vi "AVS_Main.vi"() -> ()   [LabVIEW 2016]
uses:
  Instance           5 16Saved   AVS_Main .vi
  Instance           6 16Saved   AVS_Main .vi
  Instance           4 16Saved   AVS_Main .vi
  <vilib>/express/express arith-compare/Formula/XNode/ExpressFormulaBlockNode.xnode
panel:
  out "a_hDevice":i32
  out "StartTime":u32
  out "XY Graph":cluster{"Y":dbl[], "Y":dbl[]}[](graph)
  out "LastScanTime":dbl caption="Last scan in [ms]" format="%#4.2f"
  out "AvgTimePerScan":dbl caption="Avg Time /Scan [ms]" format="%#4.2f"
  out "Failures":dbl caption="Nr Of Failures" format="%#.0f"
  out "PerformedScans":dbl caption="Nr Of Scans" format="%#.0f"
  out "TotalTime":dbl caption="Time Since Start [s]" format="%#.1f"
  in  "StopMeasurement":bool
  out "Status":string
  in  "StartMeasurement":bool caption="Start Measurement"
  in  "NrOfScans":i16 caption="Nr Of Scans"
  in  "RamSpectra":u16 caption="Spectra stored to RAM"
  in  "LaserWavelenght":sgl caption="Laser Wavelenght [nm]" format="%.2f"
  in  "LaserWidth":u32 caption="Laser Width [ns]"
  in  "LaserDelay":u32 caption="Laser Delay [ns]"
  in  "FlashesPerScan":u16 caption="Flashes per Scan"
  in  "SmoothModel":u8 caption="Model"
  in  "SmoothPix":u16 caption="Nr Of Pixels"
  in  "EnableDarkCorrection":bool caption="Enable"
  in  "DarkHist":u8 caption="%"
  in  "SatDetection":u8 caption="Saturation detection"
  in  "NrOfAVG":u32 caption="Number of averages"
  in  "IntDelay":dbl caption="Integration delay [ns]" min=-20.0 format="%#.0f"
  in  "IntTime":sgl caption="Integration time [ms]" format="%.2f"
  in  "StartPixel":u16 caption="Start pixel"
  in  "StopPixel":u16 caption="Stop pixel"
  in  "Trigger type":enum32{"Radio Selection 1", "Radio Selection 2"}(radio)
  in  "Trigger source":enum32{"Radio Selection 1", "Radio Selection 2"}(radio)
  in  "Trigger mode":T1(radio)
  out "DllVersion":string caption="AS5216 Dll Version"
  out "FWVersion":string caption="AS5216 FW Version"
  out "FPGAVersion":string caption="FPGA Version"
  out "NrOfPixel":u16 caption="Nr Of Pixels"
  out "Detector":string
  in  "Exit":bool
  in  "WriteMeasToEEProm":bool
  in  "ReadMeasFromEEProm":bool
  in  "AnalogIO":bool
  in  "DigitalIO":bool
  # "Dark Correction Settings"
  # "Measure"
  # "(-1 = infinite)"
  # "Smoothing Settings"
  # "Control Settings"
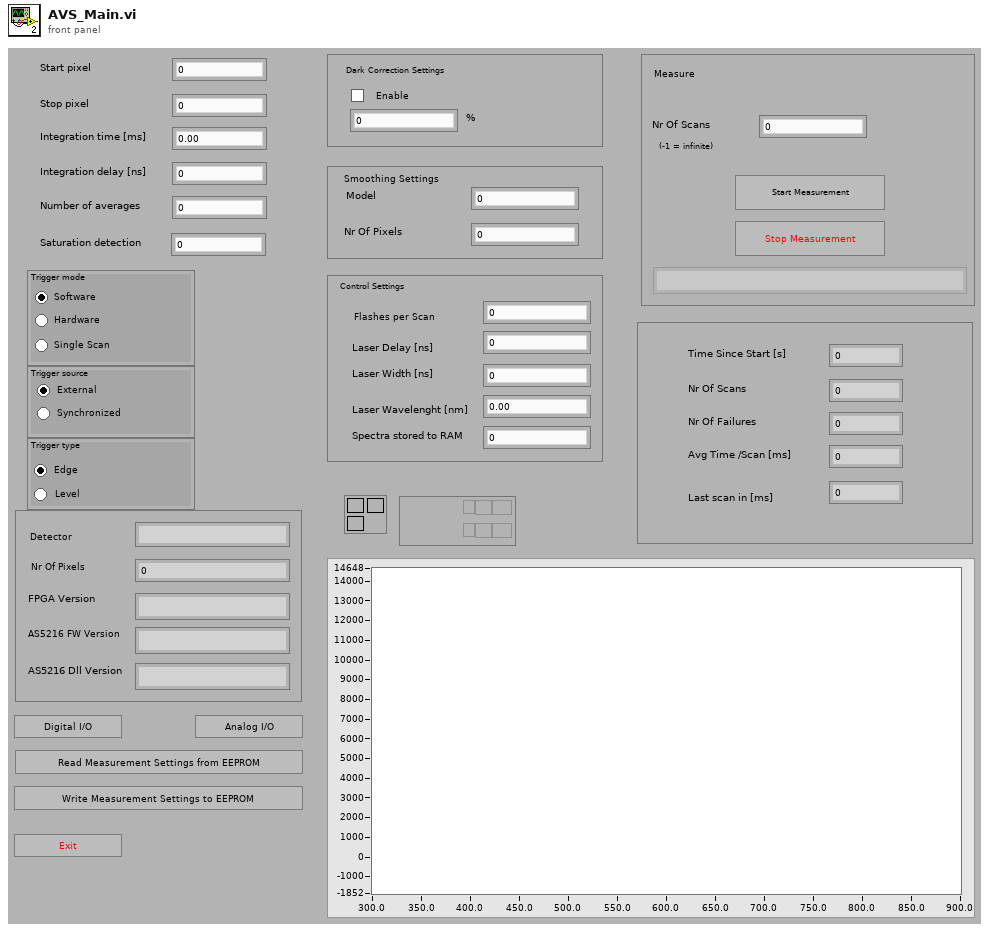
[diagram p1: front panel]
types:
  T1 = enum32{"Radio Selection 1", "Radio Selection 2", "Radio Selection 3"}
  T2 = cluster{"Len":u16, "ConfigVersion":u16, "UserFriendlyId":u8[], "DetectorType":cluster{"SensorType":u8, "NrPixels":u16, "Fit":sgl[], "NLEnable":u8, "NLCorrect":dbl[], "LowNLCounts":dbl, "HighNLCounts":dbl, "Gain":sgl[], "Reserved":sgl, "Offset":sgl[], "Extern Offset":sgl, "DefectivePixels":u16[]}, "IrradianceType":cluster{"SpectrumCalibrationType":cluster{"SmoothingType":cluster{"m_SmoothPix":u16, "SmoothModel":u8}, "CalInttime":sgl, "CalibConvers":sgl[]}, "CalibrationType":u8, "FiberDiameter":i32}, "SpectrumCalibrationType":cluster{"SmoothingType":cluster{"m_SmoothPix":u16, "SmoothModel":u8}, "CalInttime":sgl, "CalibConvers":sgl[]}, "SpectrumCorrectionType":sgl[], "StandAloneType":cluster{"StandAloneType":u8, "MeasConfigType":cluster{"StartPixel":u16, "StopPixel":u16, "IntegrationTime":sgl, "IntegrationDelay":u32, "NrAverages":u32, "DarkCorrectionType":cluster{"Enable CorDynDark":u8, "ForgetPercentage":u8}, "SmoothingType":cluster{"SmoothPix":u16, "SmoothModel":u8}, "SatDetection":u8, "TriggerType":cluster{"Trigger Mode":u8, "Trigger Source":u8, "Trigger SourceType":u8}, "ControlSettingsType":cluster{"StrobeControl":u16, "LaserDelay":u32, "LaserWidth":u32, "LaserWaveLength":sgl, "StoreToRam":u16}}, "Nmsr":i16}, "DynamicStorageType":cluster{"Nmsr":i32, "Reserved":u8[]}, "TempSensorType":sgl[], "TecControlType":cluster{"Enable":u8, "Setpoint":sgl, "Fit[NR_DAC_POL_COEF]":sgl[]}, "ProcessControlType":cluster{"AnalogLow":sgl[], "AnalogHigh":sgl[], "DigitalLow":sgl[], "DigitalHigh":sgl[]}, "EthernetSettingsType":cluster{"IpAddr":u32, "NetMask":u32, "Gateway":u32, "DhcpEnabled":u8, "TcpPort":u16, "LinkStatus":u8}, "Reserved":u8[]}
  T3 = cluster{"StartPixel":u16, "StopPixel":u16, "IntegrationTime":sgl, "IntegrationDelay":u32, "NrAverages":u32, "DarkCorrectionType":cluster{"Enable CorDynDark":u8, "ForgetPercentage":u8}, "SmoothingType":cluster{"SmoothPix":u16, "SmoothModel":u8}, "SatDetection":u8, "TriggerType":cluster{"Trigger Mode":u8, "Trigger Source":u8, "Trigger SourceType":u8}, "ControlSettingsType":cluster{"StrobeControl":u16, "LaserDelay":u32, "LaserWidth":u32, "LaserWaveLength":sgl, "StoreToRam":u16}}
  T4 = cluster{"FlashesPerScan":u16, "Result":u32, "Result":u32, "LaserWavelenght":sgl, "RamSpectra":u16}
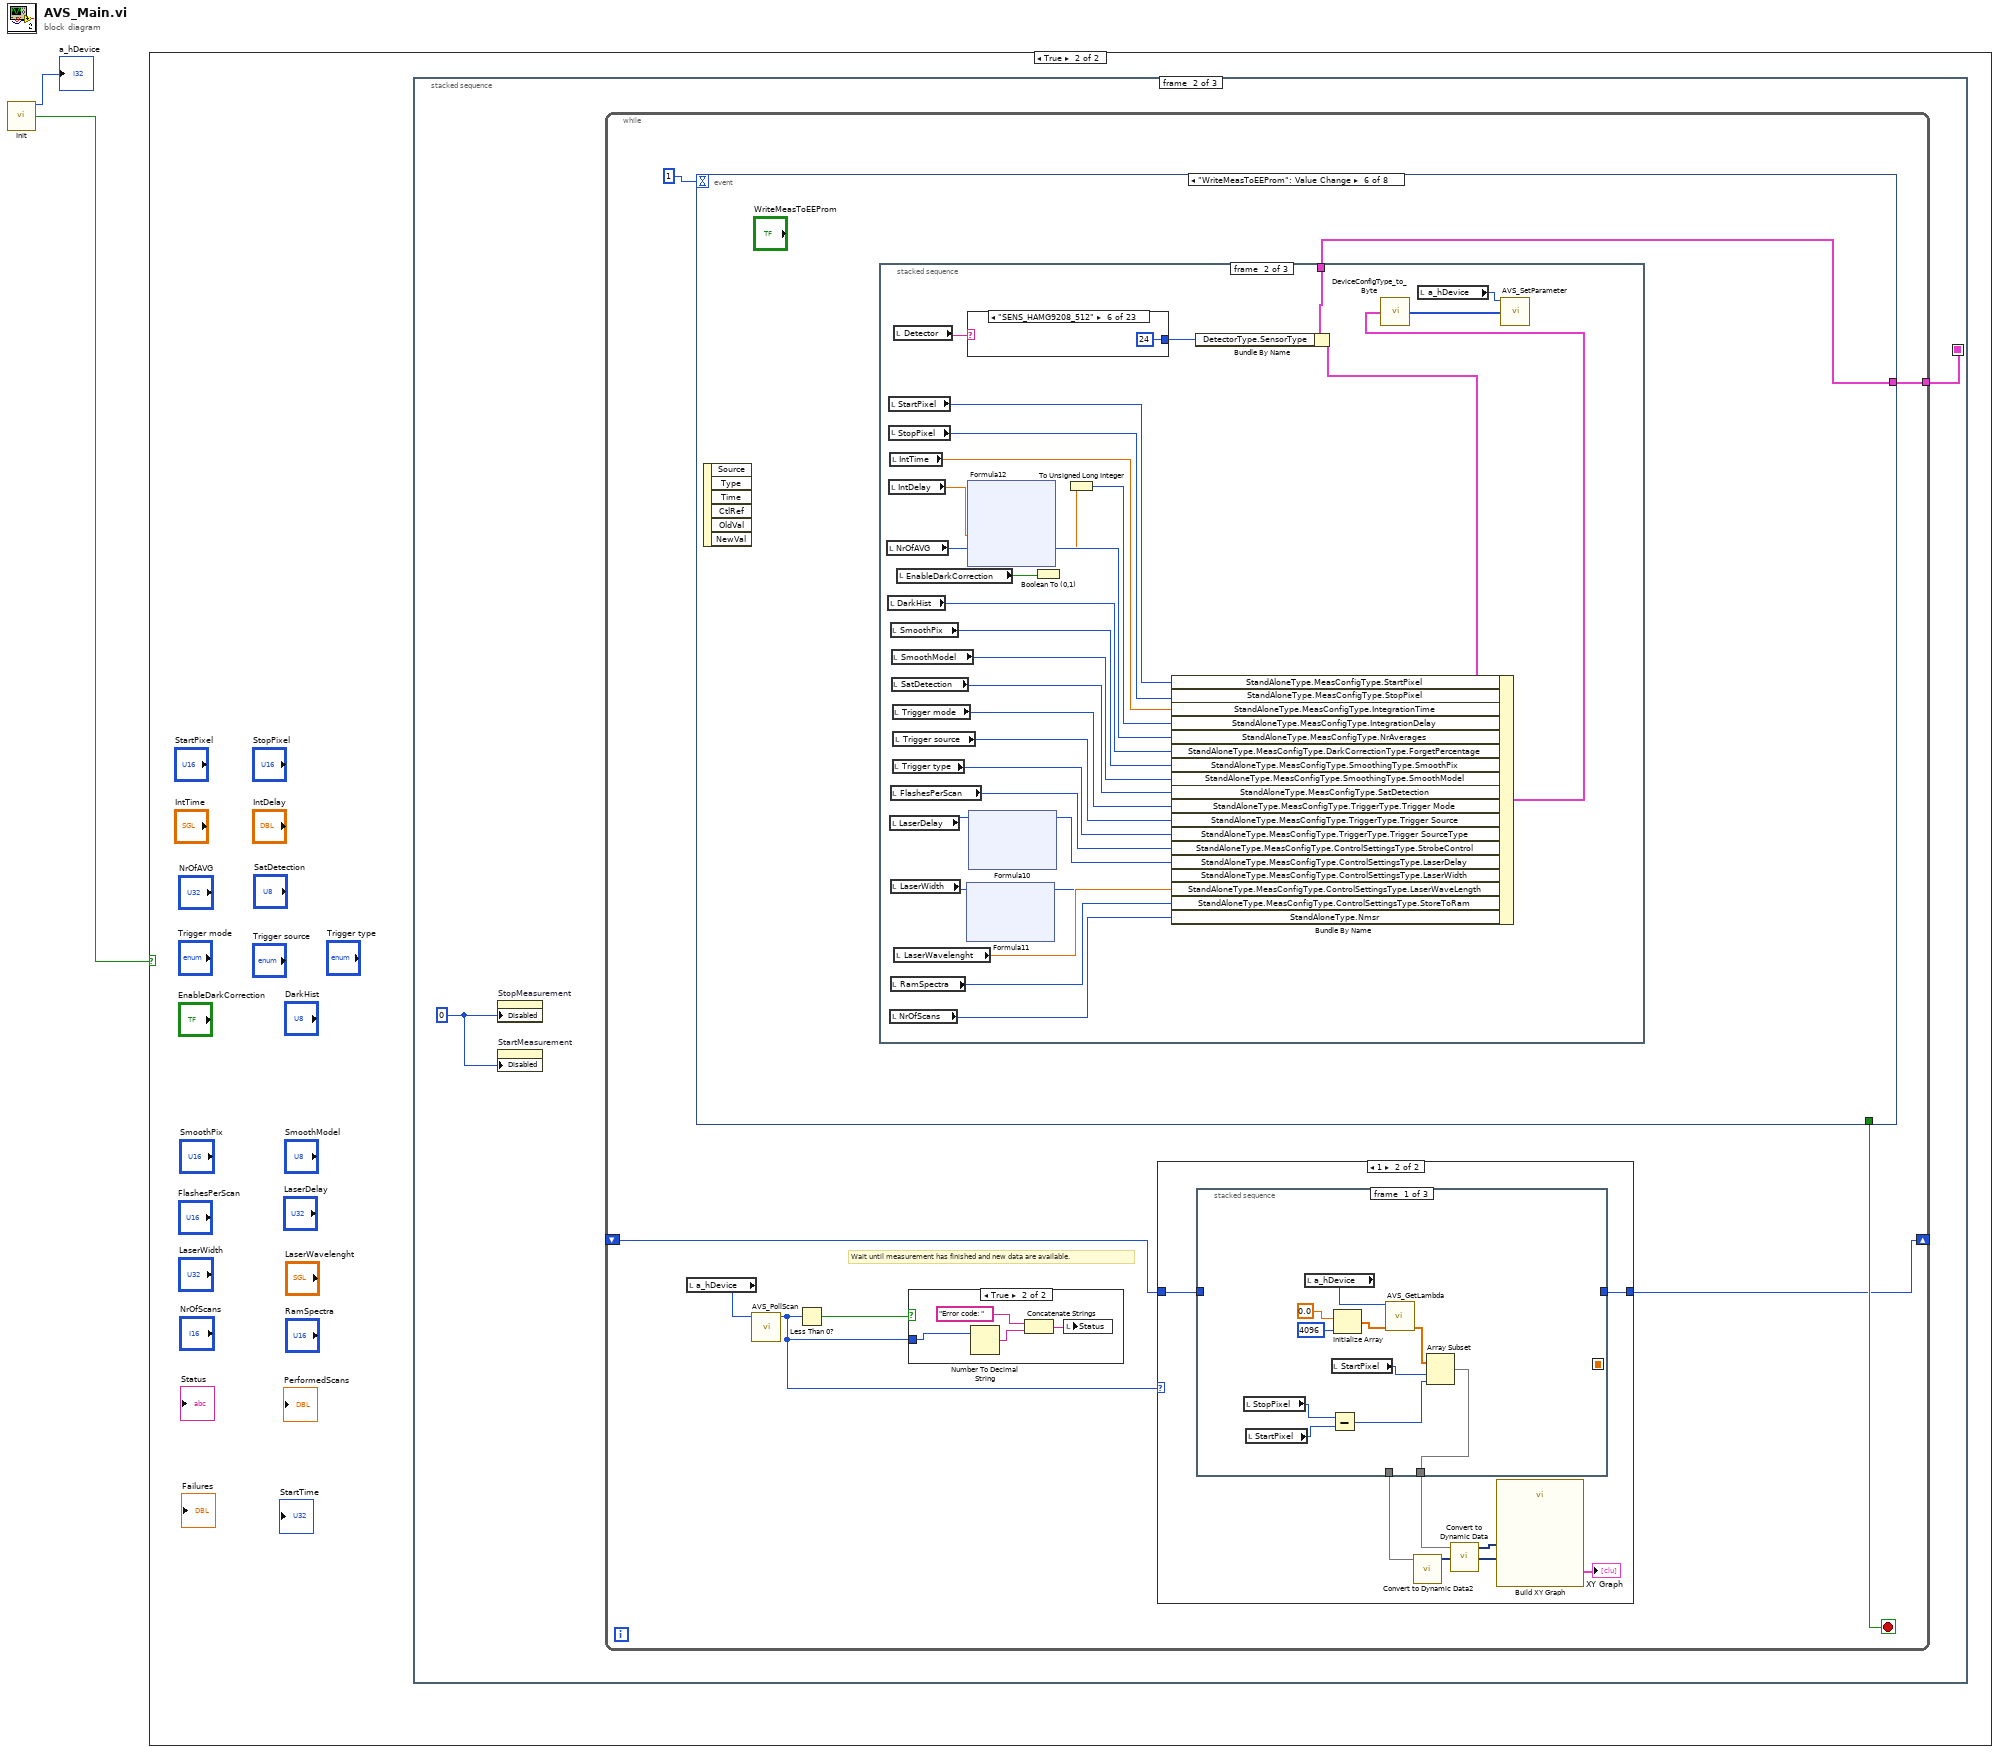
[diagram p0: block diagram]
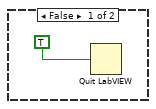
[diagram p2: hidden frame]
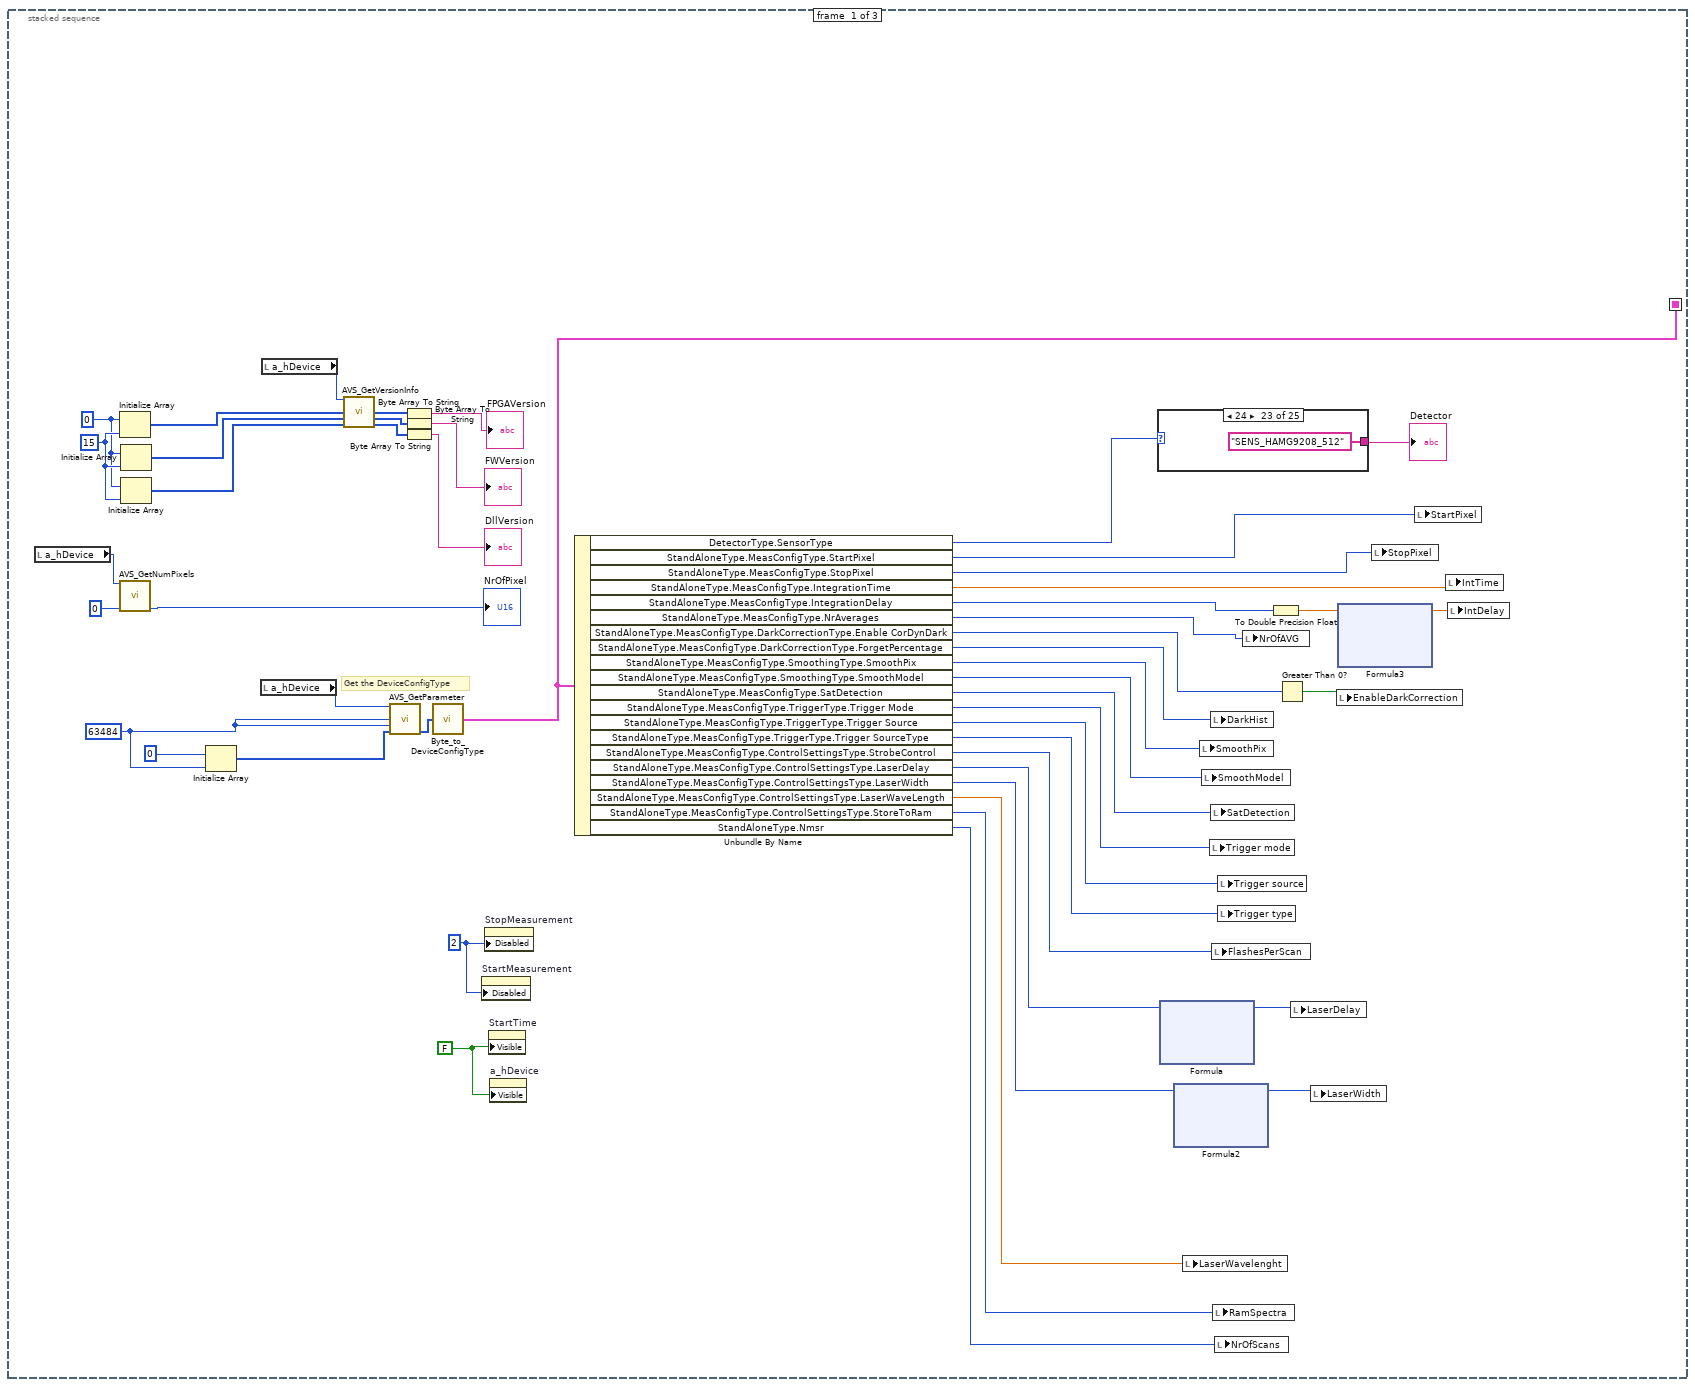
[diagram p3: hidden frame]
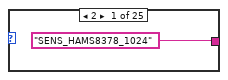
[diagram p4: hidden frame]
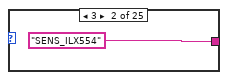
[diagram p5: hidden frame]
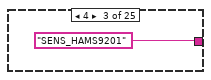
[diagram p6: hidden frame]
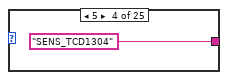
[diagram p7: hidden frame]
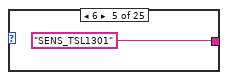
[diagram p8: hidden frame]
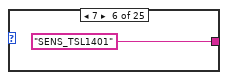
[diagram p9: hidden frame]
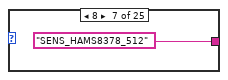
[diagram p10: hidden frame]
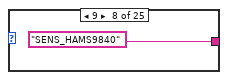
[diagram p11: hidden frame]
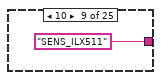
[diagram p12: hidden frame]
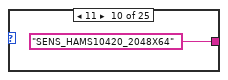
[diagram p13: hidden frame]
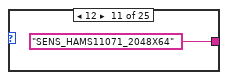
[diagram p14: hidden frame]
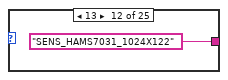
[diagram p15: hidden frame]
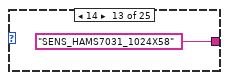
[diagram p16: hidden frame]
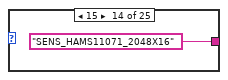
[diagram p17: hidden frame]
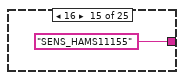
[diagram p18: hidden frame]
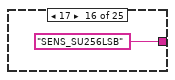
[diagram p19: hidden frame]
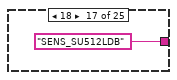
[diagram p20: hidden frame]
diagram:
  n1 = call "Init.vi"() -> ("a_hDevice"=→"a_hDevice":i32, "Available"=w2:bool)  [unwired: 14 in]
  n2 = case shown="True" w2 {
    frame False {
      n3 = Quit LabVIEW(quit? (T)=TRUE) -> ()
    }
    frame True {
      n4 = stacked-sequence {
        seq-local: [w9 _ _] -> [_ w102 _]
        frame #0 {
          w4 = FALSE
          w40 = u8 2 ("Disabled")
          w39 = u16 63484 ("a_pNumPixelsInput")
          w44 = u8 0
          w45 = u16 15 ("a_pNumPixelsInput")
          # "Get the DeviceConfigType"
          n5 = local read "a_hDevice"() -> (w8:i32)
          n6 = Initialize Array(w44, w45) -> (w48:u8[])
          n7 = call "AVS_GetNumPixels.vi"("a_hDevice"=w8, "a_pNumPixels"=u16 0 ("a_pNumPixelsInput")) -> ("a_pNumPixels"=→"NrOfPixel":u16)  [unwired: 12 in, 1 out]
          n8 = Initialize Array(w44, w45) -> (w47:u8[])
          n9 = Initialize Array(w44, w45) -> (w46:u8[])
          n10 = Initialize Array(u8 0, w39) -> (w38:u8[])
          n11 = local read "a_hDevice"() -> (w6:i32)
          n12 = local read "a_hDevice"() -> (w7:i32)
          n13 = call "AVS_GetVersionInfo.vi"("a_hDevice"=w7, "a_pFPGAVersion"=w48, "a_pFirmwareVersion"=w47, "a_pDLLVersion"=w46) -> ("a_pFPGAVersion"=w52:i8[], "a_pFirmwareVersion"=w51:i8[], "a_pDLLVersion"=w50:i8[])  [unwired: 8 in, 1 out]
          n14 = call "AVS_GetParameter.vi"("a_hDevice"=w6, "a_Size"=w39, "RequiredSizeInput"=w39, "DeviceParm"=w38) -> ("DeviceParam"=w37:u8[])  [unwired: 9 in, 2 out]
          n15 = Byte Array To String(unsigned byte array=w52) -> (string=→"FPGAVersion":string)
          n16 = Byte Array To String(unsigned byte array=w51) -> (string=→"FWVersion":string)
          n17 = Byte Array To String(unsigned byte array=w50) -> (string=→"DllVersion":string)
          n18 = call "Byte_to_DeviceConfigType.vi"("Byte Array"=w37) -> ("output cluster"=w9:T2)  [unwired: 4 in]
          n19 = property on="StartMeasurement" class="Bool"("Disabled"=w40) -> ()  [unwired: 2 in, 2 out]
          n20 = property on="StopMeasurement" class="Bool"("Disabled"=w40) -> ()  [unwired: 2 in, 2 out]
          n21 = property on="StartTime" class="DigNum (strict)"("Visible"=w4) -> ()  [unwired: 2 in, 2 out]
          n22 = property on="a_hDevice" class="DigNum (strict)"("Visible"=w4) -> ()  [unwired: 2 in, 2 out]
          n23 = Unbundle By Name(w9) -> ("DetectorType.SensorType"=w34:u8, "StandAloneType.MeasConfigType.StartPixel"=w33:u16, "StandAloneType.MeasConfigType.StopPixel"=w32:u16, "StandAloneType.MeasConfigType.IntegrationTime"=w31:sgl, "StandAloneType.MeasConfigType.IntegrationDelay"=w30:u32, "StandAloneType.MeasConfigType.NrAverages"=w29:u32, "StandAloneType.MeasConfigType.DarkCorrectionType.Enable CorDynDark"=w27:u8, "StandAloneType.MeasConfigType.DarkCorrectionType.ForgetPercentage"=w26:u8, "StandAloneType.MeasConfigType.SmoothingType.SmoothPix"=w25:u16, "StandAloneType.MeasConfigType.SmoothingType.SmoothModel"=w24:u8, "StandAloneType.MeasConfigType.SatDetection"=w23:u8, "StandAloneType.MeasConfigType.TriggerType.Trigger Mode"=w22:u8, "StandAloneType.MeasConfigType.TriggerType.Trigger Source"=w21:u8, "StandAloneType.MeasConfigType.TriggerType.Trigger SourceType"=w20:u8, "StandAloneType.MeasConfigType.ControlSettingsType.StrobeControl"=w19:u16, "StandAloneType.MeasConfigType.ControlSettingsType.LaserDelay"=w18:u32, "StandAloneType.MeasConfigType.ControlSettingsType.LaserWidth"=w17:u32, "StandAloneType.MeasConfigType.ControlSettingsType.LaserWaveLength"=w16:sgl, "StandAloneType.MeasConfigType.ControlSettingsType.StoreToRam"=w15:u16, "StandAloneType.Nmsr"=w14:i16)
          n24 = case shown="24" w34 {
            tunnel: ["SENS_HAMS8378_1024" ("String") "SENS_ILX554" ("String") "SENS_HAMS9201" ("String") "SENS_TCD1304" ("String") "SENS_TSL1301" ("String") "SENS_TSL1401" ("String") "SENS_HAMS8378_512" ("String") "SENS_HAMS9840" ("String") "SENS_ILX511" ("String") "SENS_HAMS10420_2048X64" ("String") "SENS_HAMS11071_2048X64" ("String") "SENS_HAMS7031_1024X122" ("String") "SENS_HAMS7031_1024X58" ("String") "SENS_HAMS11071_2048X16" ("String") "SENS_HAMS11155" ("String") "SENS_SU256LSB" ("String") "SENS_SU512LDB" ("String") "unknown" ("String") "unknown" ("String") "SENS_HAMS11638" ("String") "SENS_HAMS11639" ("String") "SENS_HAMS12443" ("String") "SENS_HAMG9208_512" ("String") "unknown" ("String") "SENS_HAMS8378_256" ("String")] -> w5
            frame 2 {
            }
            frame 3 {
            }
            frame 4 {
            }
            frame 5 {
            }
            frame 6 {
            }
            frame 7 {
            }
            frame 8 {
            }
            frame 9 {
            }
            frame 10 {
            }
            frame 11 {
            }
            frame 12 {
            }
            frame 13 {
            }
            frame 14 {
            }
            frame 15 {
            }
            frame 16 {
            }
            frame 17 {
            }
            frame 18 {
            }
            frame 19 {
            }
            frame 20 {
            }
            frame 21 {
            }
            frame 22 {
            }
            frame 23 {
            }
            frame 24 {
            }
            frame Default {
            }
            frame 1 {
            }
          }
          "Detector" <- w5
          n25 = xnode "Formula"("X1"=w18) -> ("Result"=w42:u32)  [unwired: 1 in, 1 out]
          n26 = xnode "Formula2"("X1"=w17) -> ("Result"=w41:u32)  [unwired: 1 in, 1 out]
          n27 = local write "LaserWavelenght"(w16) -> ()
          n28 = local write "SmoothPix"(w25) -> ()
          n29 = local write "SmoothModel"(w24) -> ()
          n30 = local write "Trigger mode"(w22) -> ()
          n31 = local write "DarkHist"(w26) -> ()
          n32 = local write "SatDetection"(w23) -> ()
          n33 = local write "FlashesPerScan"(w19) -> ()
          n34 = local write "RamSpectra"(w15) -> ()
          n35 = local write "NrOfScans"(w14) -> ()
          n36 = local write "Trigger source"(w21) -> ()
          n37 = local write "Trigger type"(w20) -> ()
          n38 = local write "NrOfAVG"(w29) -> ()
          n39 = To Double Precision Float(number=w30) -> (double precision float=w36:dbl)
          n40 = Greater Than 0?(x=w27) -> (x > 0?=w28:bool)
          n41 = local write "LaserDelay"(w42) -> ()
          n42 = local write "LaserWidth"(w41) -> ()
          n43 = local write "EnableDarkCorrection"(w28) -> ()
          n44 = xnode "Formula3"("X1"=w36) -> ("Result"=w35:dbl)  [unwired: 1 in, 1 out]
          n45 = local write "StopPixel"(w32) -> ()
          n46 = local write "StartPixel"(w33) -> ()
          n47 = local write "IntTime"(w31) -> ()
          n48 = local write "IntDelay"(w35) -> ()
        }
        frame #1 {
          w103 = u8 0 ("Disabled")
          n49 = property on="StopMeasurement" class="Bool"("Disabled"=w103) -> ()  [unwired: 2 in, 2 out]
          n50 = property on="StartMeasurement" class="Bool"("Disabled"=w103) -> ()  [unwired: 2 in, 2 out]
          n51 = while {
            tunnel: w102 -> [w107]
            shift-right: [w106] -> _
            shift-left: _ -> [w105]
            stop <- w111 stop-if-true
            # "Wait until measurement has finished and new data are available."
            n52 = local read "a_hDevice"() -> (w109:i32)
            n53 = event shown="[5] \"WriteMeasToEEProm\": Value Change" {
              selector: _ -> [_ _ _ _ _ _ _ _]
              dyn-events: _ -> [_ _ _ _ _ _ _ _]
              timeout: 1 -> [_ _ _ _ _ _ _ _]
              tunnel: [_ _ _ _ _ _ _ "Exit"] -> w111
              tunnel: w107 -> [_ _ _ _ _ w320 _ _]
              event Timeout {
                n54 = event-data() -> ()  [unwired: 1 in, 2 out]
              }
              event "StartMeasurement": Value Change {
                w190 = T3 {"StartPixel"=0, "StopPixel"=0, "IntegrationTime"=0.0, "IntegrationDelay"=0, "NrAverages"=0, "DarkCorrectionType"={"Enable CorDynDark"=0, "ForgetPercentage"=0}, "SmoothingType"={"SmoothPix"=0, "SmoothModel"=0}, "SatDetection"=0, "TriggerType"={"Trigger Mode"=0, "Trigger Source"=0, "Trigger SourceType"=0}, "ControlSettingsType"={"StrobeControl"=0, "LaserDelay"=0, "LaserWidth"=0, "LaserWaveLength"=0.0, "StoreToRam"=0}}  # MeasConfigType
                w172 = u8 2 ("Disabled")
                w196 = 0.0 ("Failures")
                # "StartMeas:\n1: Prepares measurement on the spectrometer \nusing the specified measurement configuration. \n2: Start measurement"
                n55 = event-data() -> ()  [unwired: 1 in, 6 out]
                n56 = local read "EnableDarkCorrection"() -> (w197:bool)
                n57 = local read "SmoothModel"() -> (w185:u8)
                n58 = local read "Trigger mode"() -> (w199:T1)
                n59 = local read "FlashesPerScan"() -> (w173:u16)
                n60 = local read "SmoothPix"() -> (w186:u16)
                n61 = local read "SatDetection"() -> (w182:u8)
                n62 = local read "RamSpectra"() -> (w177:u16)
                n63 = local read "Trigger source"() -> (w200:enum32{"Radio Selection 1", "Radio Selection 2"})
                n64 = local read "LaserWavelenght"() -> (w176:sgl)
                n65 = local read "DarkHist"() -> (w188:u8)
                n66 = local read "Trigger type"() -> (w198:enum32{"Radio Selection 1", "Radio Selection 2"})
                n67 = local read "LaserDelay"() -> (w192:u32)
                n68 = local read "LaserWidth"() -> (w191:u32)
                n69 = local read "StartPixel"() -> (w204:u16)
                n70 = local read "StopPixel"() -> (w203:u16)
                n71 = local read "IntTime"() -> (w202:sgl)
                n72 = local read "NrOfAVG"() -> (w205:u32)
                n73 = local read "IntDelay"() -> (w193:dbl)
                n74 = xnode "Formula6"("X1"=w191) -> ("Result"=w175:u32)  [unwired: 1 in, 1 out]
                n75 = xnode "Formula5"("X1"=w192) -> ("Result"=w174:u32)  [unwired: 1 in, 1 out]
                n76 = Boolean To (0,1)(Boolean=w197) -> (0, 1=w201:i16)
                n77 = Bundle("SmoothPix"=w186, "SmoothModel"=w185) -> (w184:cluster{"SmoothPix":u16, "SmoothModel":u8})  [unwired: 1 in]
                n78 = xnode "Formula4"("X1"=w193) -> ("Result"=w194:dbl)  [unwired: 1 in, 1 out]
                n79 = To Unsigned Byte Integer(number=w201) -> (unsigned 8bit integer=w189:u8)
                n80 = To Unsigned Byte Integer(number=w200) -> (unsigned 8bit integer=w180:u8)
                n81 = Bundle(w189, "DarkHist"=w188) -> (w187:cluster{u8, "DarkHist":u8})  [unwired: 1 in]
                n82 = To Unsigned Byte Integer(number=w199) -> (unsigned 8bit integer=w183:u8)
                n83 = To Unsigned Byte Integer(number=w198) -> (unsigned 8bit integer=w181:u8)
                n84 = To Unsigned Long Integer(number=w194) -> (unsigned 32bit integer=w195:u32)
                n85 = Bundle("FlashesPerScan"=w173, "Result"=w174, "Result"=w175, "LaserWavelenght"=w176, "RamSpectra"=w177) -> (w178:T4)  [unwired: 1 in]
                n86 = Bundle(w183, w180, w181) -> (w179:cluster{u8, u8, u8})  [unwired: 1 in]
                n87 = Bundle(cluster=w190, "StartPixel"=w204, "StopPixel"=w203, "IntegrationTime"=w202, "IntegrationDelay"=w195, "NrAverages"=w205, "DarkCorrectionType"=w187, "SmoothingType"=w184, "SatDetection"=w182, "TriggerType"=w179, "ControlSettingsType"=w178) -> (w206:T3)
                n88 = local write "Failures"(w196) -> ()
                n89 = local write "TotalTime"(w196) -> ()
                n90 = local write "PerformedScans"(w196) -> ()
                n91 = local write "AvgTimePerScan"(w196) -> ()
                n92 = local write "LastScanTime"(w196) -> ()
                n93 = local read "NrOfScans"() -> (w168:i16)
                n94 = local read "a_hDevice"() -> (w169:i32)
                n95 = call "StartMeasurement.vi"("a_hDevice"=w169, "a_hWnd"=0, "a_Nmsr"=w168, "MeasConfigType"=w206) -> ("Status"=w171:string, "StartTime"=w170:u32)  [unwired: 10 in]
                n96 = local write "StartTime"(w170) -> ()
                n97 = local write "Status"(w171) -> ()
                n98 = property on="StartMeasurement" class="Bool"("Disabled"=w172) -> ()  [unwired: 2 in, 2 out]
                n99 = property on="AnalogIO" class="Bool"("Disabled"=w172) -> ()  [unwired: 2 in, 2 out]
                n100 = property on="DigitalIO" class="Bool"("Disabled"=w172) -> ()  [unwired: 2 in, 2 out]
                n101 = property on="ReadMeasFromEEProm" class="Bool"("Disabled"=w172) -> ()  [unwired: 2 in, 2 out]
                n102 = property on="WriteMeasToEEProm" class="Bool"("Disabled"=w172) -> ()  [unwired: 2 in, 2 out]
              }
              event "AnalogIO": Value Change {
                n103 = event-data() -> ()  [unwired: 1 in, 6 out]
                n104 = flat-sequence {
                  frame #0 {
                    w231 = u8 2 ("Disabled")
                    n105 = property on="StopMeasurement" class="Bool"("Disabled"=w231) -> ()  [unwired: 2 in, 2 out]
                    n106 = property on="StartMeasurement" class="Bool"("Disabled"=w231) -> ()  [unwired: 2 in, 2 out]
                    n107 = property on="DigitalIO" class="Bool"("Disabled"=w231) -> ()  [unwired: 2 in, 2 out]
                    n108 = property on="ReadMeasFromEEProm" class="Bool"("Disabled"=w231) -> ()  [unwired: 2 in, 2 out]
                    n109 = property on="WriteMeasToEEProm" class="Bool"("Disabled"=w231) -> ()  [unwired: 2 in, 2 out]
                  }
                  frame #1 {
                    n110 = local read "a_hDevice"() -> (w232:i32)
                    n111 = call "AnalogIO.vi"("a_hDevice"=w232) -> ()  [unwired: 15 in]
                  }
                  frame #2 {
                    w233 = u8 0 ("Disabled")
                    n112 = property on="StopMeasurement" class="Bool"("Disabled"=w233) -> ()  [unwired: 2 in, 2 out]
                    n113 = property on="StartMeasurement" class="Bool"("Disabled"=w233) -> ()  [unwired: 2 in, 2 out]
                    n114 = property on="DigitalIO" class="Bool"("Disabled"=w233) -> ()  [unwired: 2 in, 2 out]
                    n115 = property on="ReadMeasFromEEProm" class="Bool"("Disabled"=w233) -> ()  [unwired: 2 in, 2 out]
                    n116 = property on="WriteMeasToEEProm" class="Bool"("Disabled"=w233) -> ()  [unwired: 2 in, 2 out]
                  }
                }
              }
              event "DigitalIO": Value Change {
                n117 = event-data() -> ()  [unwired: 1 in, 6 out]
                n118 = flat-sequence {
                  frame #0 {
                    w234 = u8 2 ("Disabled")
                    n119 = property on="StartMeasurement" class="Bool"("Disabled"=w234) -> ()  [unwired: 2 in, 2 out]
                    n120 = property on="StopMeasurement" class="Bool"("Disabled"=w234) -> ()  [unwired: 2 in, 2 out]
                    n121 = property on="AnalogIO" class="Bool"("Disabled"=w234) -> ()  [unwired: 2 in, 2 out]
                    n122 = property on="WriteMeasToEEProm" class="Bool"("Disabled"=w234) -> ()  [unwired: 2 in, 2 out]
                    n123 = property on="ReadMeasFromEEProm" class="Bool"("Disabled"=w234) -> ()  [unwired: 2 in, 2 out]
                  }
                  frame #1 {
                    n124 = local read "a_hDevice"() -> (w235:i32)
                    n125 = call "DigitalIO.vi"("a_hDevice"=w235) -> ()  [unwired: 15 in]
                  }
                  frame #2 {
                    w236 = u8 0 ("Disabled")
                    n126 = property on="StopMeasurement" class="Bool"("Disabled"=w236) -> ()  [unwired: 2 in, 2 out]
                    n127 = property on="StartMeasurement" class="Bool"("Disabled"=w236) -> ()  [unwired: 2 in, 2 out]
                    n128 = property on="AnalogIO" class="Bool"("Disabled"=w236) -> ()  [unwired: 2 in, 2 out]
                    n129 = property on="ReadMeasFromEEProm" class="Bool"("Disabled"=w236) -> ()  [unwired: 2 in, 2 out]
                    n130 = property on="WriteMeasToEEProm" class="Bool"("Disabled"=w236) -> ()  [unwired: 2 in, 2 out]
                  }
                }
              }
              event "ReadMeasFromEEProm": Value Change {
                n131 = event-data() -> ()  [unwired: 1 in, 6 out]
                n132 = stacked-sequence {
                  frame #0 {
                    w237 = u8 2 ("Disabled")
                    n133 = property on="StartMeasurement" class="Bool"("Disabled"=w237) -> ()  [unwired: 2 in, 2 out]
                    n134 = property on="StopMeasurement" class="Bool"("Disabled"=w237) -> ()  [unwired: 2 in, 2 out]
                    n135 = property on="AnalogIO" class="Bool"("Disabled"=w237) -> ()  [unwired: 2 in, 2 out]
                    n136 = property on="WriteMeasToEEProm" class="Bool"("Disabled"=w237) -> ()  [unwired: 2 in, 2 out]
                    n137 = property on="DigitalIO" class="Bool"("Disabled"=w237) -> ()  [unwired: 2 in, 2 out]
                  }
                  frame #1 {
                    w269 = u16 63484 ("a_pNumPixelsInput")
                    n138 = local read "a_hDevice"() -> (w238:i32)
                    n139 = Initialize Array(u8 0, w269) -> (w268:u8[])
                    n140 = call "AVS_GetParameter.vi"("a_hDevice"=w238, "a_Size"=w269, "RequiredSizeInput"=w269, "DeviceParm"=w268) -> ("DeviceParam"=w260:u8[])  [unwired: 9 in, 2 out]
                    n141 = call "Byte_to_DeviceConfigType.vi"("Byte Array"=w260) -> ("output cluster"=w239:T2)  [unwired: 4 in]
                    n142 = Unbundle By Name(w239) -> ("DetectorType.SensorType"=w259:u8, "StandAloneType.MeasConfigType.StartPixel"=w258:u16, "StandAloneType.MeasConfigType.StopPixel"=w257:u16, "StandAloneType.MeasConfigType.IntegrationTime"=w256:sgl, "StandAloneType.MeasConfigType.IntegrationDelay"=w255:u32, "StandAloneType.MeasConfigType.NrAverages"=w254:u32, "StandAloneType.MeasConfigType.DarkCorrectionType.Enable CorDynDark"=w252:u8, "StandAloneType.MeasConfigType.DarkCorrectionType.ForgetPercentage"=w251:u8, "StandAloneType.Nmsr"=w253:i16, "StandAloneType.MeasConfigType.SmoothingType.SmoothPix"=w250:u16, "StandAloneType.MeasConfigType.SmoothingType.SmoothModel"=w249:u8, "StandAloneType.MeasConfigType.SatDetection"=w248:u8, "StandAloneType.MeasConfigType.TriggerType.Trigger Mode"=w247:u8, "StandAloneType.MeasConfigType.TriggerType.Trigger Source"=w246:u8, "StandAloneType.MeasConfigType.TriggerType.Trigger SourceType"=w245:u8, "StandAloneType.MeasConfigType.ControlSettingsType.StrobeControl"=w240:u16, "StandAloneType.MeasConfigType.ControlSettingsType.LaserDelay"=w241:u32, "StandAloneType.MeasConfigType.ControlSettingsType.LaserWidth"=w242:u32, "StandAloneType.MeasConfigType.ControlSettingsType.LaserWaveLength"=w243:sgl, "StandAloneType.MeasConfigType.ControlSettingsType.StoreToRam"=w244:u16)
                    n143 = case shown="24" w259 {
                      tunnel: ["SENS_HAMS8378_1024" ("String") "SENS_ILX554" ("String") "SENS_HAMS9201" ("String") "SENS_TCD1304" ("String") "SENS_TSL1301" ("String") "SENS_TSL1401" ("String") "SENS_HAMS8378_512" ("String") "SENS_HAMS9840" ("String") "SENS_ILX511" "SENS_HAMS10420_2048X64" ("String") "SENS_HAMS11071_2048X64" ("String") "SENS_HAMS7031_1024X122" ("String") "SENS_HAMS7031_1024X58" ("String") "SENS_HAMS11071_2048X16" ("String") "SENS_HAMS11155" ("String") "SENS_SU256LSB" ("String") "SENS_SU512LDB" ("String") "unknown" ("String") "unknown" ("String") "SENS_HAMS11638" ("String") "SENS_HAMS11639" ("String") "SENS_HAMS12443" ("String") "SENS_HAMG9208_512" ("String") "unknown" ("String") "SENS_HAMS8378_256" ("String")] -> w266
                      frame 2 {
                      }
                      frame 3 {
                      }
                      frame 4 {
                      }
                      frame 5 {
                      }
                      frame 6 {
                      }
                      frame 7 {
                      }
                      frame 8 {
                      }
                      frame 9 {
                      }
                      frame 10 {
                      }
                      frame 11 {
                      }
                      frame 12 {
                      }
                      frame 13 {
                      }
                      frame 14 {
                      }
                      frame 15 {
                      }
                      frame 16 {
                      }
                      frame 17 {
                      }
                      frame 18 {
                      }
                      frame 19 {
                      }
                      frame 20 {
                      }
                      frame 21 {
                      }
                      frame 22 {
                      }
                      frame 23 {
                      }
                      frame 24 {
                      }
                      frame Default {
                      }
                      frame 1 {
                      }
                    }
                    n144 = To Double Precision Float(number=w255) -> (double precision float=w261:dbl)
                    n145 = local write "IntTime"(w256) -> ()
                    n146 = local write "Trigger mode"(w247) -> ()
                    n147 = local write "NrOfAVG"(w254) -> ()
                    n148 = xnode "Formula7"("X1"=w241) -> ("Result"=w263:u32)  [unwired: 1 in, 1 out]
                    n149 = xnode "Formula8"("X1"=w242) -> ("Result"=w262:u32)  [unwired: 1 in, 1 out]
                    n150 = local write "Trigger type"(w245) -> ()
                    n151 = local write "FlashesPerScan"(w240) -> ()
                    n152 = local write "RamSpectra"(w244) -> ()
                    n153 = local write "LaserWavelenght"(w243) -> ()
                    n154 = local write "SmoothPix"(w250) -> ()
                    n155 = local write "NrOfScans"(w253) -> ()
                    n156 = local write "SatDetection"(w248) -> ()
                    n157 = Greater Than 0?(x=w252) -> (x > 0?=w265:bool)
                    n158 = xnode "Formula9"("X1"=w261) -> ("Result"=w264:dbl)  [unwired: 1 in, 1 out]
                    n159 = local write "EnableDarkCorrection"(w265) -> ()
                    n160 = local write "StopPixel"(w257) -> ()
                    n161 = local write "StartPixel"(w258) -> ()
                    n162 = local write "SmoothModel"(w249) -> ()
                    n163 = local write "Trigger source"(w246) -> ()
                    n164 = local write "DarkHist"(w251) -> ()
                    n165 = local write "LaserDelay"(w263) -> ()
                    n166 = local write "LaserWidth"(w262) -> ()
                    n167 = local write "IntDelay"(w264) -> ()
                    n168 = local write "Detector"(w266) -> ()
                  }
                  frame #2 {
                    w319 = u8 0 ("Disabled")
                    n169 = property on="StopMeasurement" class="Bool"("Disabled"=w319) -> ()  [unwired: 2 in, 2 out]
                    n170 = property on="AnalogIO" class="Bool"("Disabled"=w319) -> ()  [unwired: 2 in, 2 out]
                    n171 = property on="DigitalIO" class="Bool"("Disabled"=w319) -> ()  [unwired: 2 in, 2 out]
                    n172 = property on="StartMeasurement" class="Bool"("Disabled"=w319) -> ()  [unwired: 2 in, 2 out]
                    n173 = property on="WriteMeasToEEProm" class="Bool"("Disabled"=w319) -> ()  [unwired: 2 in, 2 out]
                  }
                }
              }
              event "WriteMeasToEEProm": Value Change {
                n174 = event-data() -> ()  [unwired: 1 in, 6 out]
                n175 = stacked-sequence {
                  tunnel: w320 -> [_ w323 _]
                  frame #0 {
                    w321 = u8 2 ("Disabled")
                    n176 = property on="StopMeasurement" class="Bool"("Disabled"=w321) -> ()  [unwired: 2 in, 2 out]
                    n177 = property on="ReadMeasFromEEProm" class="Bool"("Disabled"=w321) -> ()  [unwired: 2 in, 2 out]
                    n178 = property on="AnalogIO" class="Bool"("Disabled"=w321) -> ()  [unwired: 2 in, 2 out]
                    n179 = property on="DigitalIO" class="Bool"("Disabled"=w321) -> ()  [unwired: 2 in, 2 out]
                    n180 = property on="StartMeasurement" class="Bool"("Disabled"=w321) -> ()  [unwired: 2 in, 2 out]
                  }
                  frame #1 {
                    n181 = local read "NrOfAVG"() -> (w334:u32)
                    n182 = local read "DarkHist"() -> (w336:u8)
                    n183 = local read "StartPixel"() -> (w330:u16)
                    n184 = local read "StopPixel"() -> (w331:u16)
                    n185 = local read "IntDelay"() -> (w333:dbl)
                    n186 = local read "IntTime"() -> (w332:sgl)
                    n187 = local read "LaserDelay"() -> (w344:u32)
                    n188 = local read "NrOfScans"() -> (w350:i16)
                    n189 = local read "SmoothPix"() -> (w337:u16)
                    n190 = local read "FlashesPerScan"() -> (w343:u16)
                    n191 = local read "LaserWidth"() -> (w345:u32)
                    n192 = local read "RamSpectra"() -> (w349:u16)
                    n193 = local read "SmoothModel"() -> (w338:u8)
                    n194 = local read "SatDetection"() -> (w339:u8)
                    n195 = local read "Trigger mode"() -> (w340:T1)
                    n196 = local read "Trigger type"() -> (w342:enum32{"Radio Selection 1", "Radio Selection 2"})
                    n197 = local read "Trigger source"() -> (w341:enum32{"Radio Selection 1", "Radio Selection 2"})
                    n198 = local read "Detector"() -> (w329:string)
                    n199 = local read "LaserWavelenght"() -> (w348:sgl)
                    n200 = local read "EnableDarkCorrection"() -> (w335:bool)
                    n201 = xnode "Formula11"("X1"=w345) -> ("Result"=w347:u32)  [unwired: 1 in, 1 out]
                    n202 = case shown="\"SENS_HAMG9208_512\"" w329 {
                      tunnel: [2 3 21 22 23 24 4 5 6 7 8 9 10 11 12 13 14 15 16 17 18 0 1] -> w325
                      frame "SENS_HAMS8378_1024" {
                      }
                      frame "SENS_ILX554" {
                      }
                      frame "SENS_HAMS11638" {
                      }
                      frame "SENS_HAMS11639" {
                      }
                      frame "SENS_HAMS12443" {
                      }
                      frame "SENS_HAMG9208_512" {
                      }
                      frame "SENS_HAMS9201" {
                      }
                      frame "SENS_TCD1304" {
                      }
                      frame "SENS_TSL1301" {
                      }
                      frame "SENS_TSL1401" {
                      }
                      frame "SENS_HAMS8378_512" {
                      }
                      frame "SENS_HAMS9840" {
                      }
                      frame "SENS_ILX511" {
                      }
                      frame "SENS_HAMS10420_2048X64" {
                      }
                      frame "SENS_HAMS11071_2048X64" {
                      }
                      frame "SENS_HAMS7031_1024X122" {
                      }
                      frame "SENS_HAMS7031_1024X58" {
                      }
                      frame "SENS_HAMS11071_2048X16" {
                      }
                      frame "SENS_HAMS11155" {
                      }
                      frame "SENS_SU256LSB" {
                      }
                      frame "SENS_SU512LDB" {
                      }
                      frame Default {
                      }
                      frame "SENS_HAMS8378_256" {
                      }
                    }
                    n203 = xnode "Formula12"("X1"=w333) -> ("Result"=w328:dbl)  [unwired: 1 in, 1 out]
                    n204 = xnode "Formula10"("X1"=w344) -> ("Result"=w346:u32)  [unwired: 1 in, 1 out]
                    n205 = Boolean To (0,1)(Boolean=w335) -> ()  [unwired: 1 out]
                    n206 = To Unsigned Long Integer(number=w328) -> (unsigned 32bit integer=w327:u32)
                    n207 = Bundle By Name(cluster=w323, "DetectorType.SensorType"=w325) -> (w326:T2)
                    n208 = Bundle By Name(cluster=w326, "StandAloneType.MeasConfigType.StartPixel"=w330, "StandAloneType.MeasConfigType.StopPixel"=w331, "StandAloneType.MeasConfigType.IntegrationTime"=w332, "StandAloneType.MeasConfigType.IntegrationDelay"=w327, "StandAloneType.MeasConfigType.NrAverages"=w334, "StandAloneType.MeasConfigType.DarkCorrectionType.ForgetPercentage"=w336, "StandAloneType.MeasConfigType.SmoothingType.SmoothPix"=w337, "StandAloneType.MeasConfigType.SmoothingType.SmoothModel"=w338, "StandAloneType.MeasConfigType.SatDetection"=w339, "StandAloneType.MeasConfigType.TriggerType.Trigger Mode"=w340, "StandAloneType.MeasConfigType.TriggerType.Trigger Source"=w341, "StandAloneType.MeasConfigType.TriggerType.Trigger SourceType"=w342, "StandAloneType.MeasConfigType.ControlSettingsType.StrobeControl"=w343, "StandAloneType.MeasConfigType.ControlSettingsType.LaserDelay"=w346, "StandAloneType.MeasConfigType.ControlSettingsType.LaserWidth"=w347, "StandAloneType.MeasConfigType.ControlSettingsType.LaserWaveLength"=w348, "StandAloneType.MeasConfigType.ControlSettingsType.StoreToRam"=w349, "StandAloneType.Nmsr"=w350) -> (w322:T2)
                    n209 = call "DeviceConfigType_to_Byte.vi"("DeviceConfig"=w322) -> ("Byte Array"=w351:u8[])  [unwired: 4 in]
                    n210 = local read "a_hDevice"() -> (w324:i32)
                    n211 = call "AVS_SetParameter.vi"("a_hDevice"=w324, "a_pDeviceParm"=w351) -> ()  [unwired: 12 in, 2 out]
                  }
                  frame #2 {
                    w399 = u8 0 ("Disabled")
                    n212 = property on="StopMeasurement" class="Bool"("Disabled"=w399) -> ()  [unwired: 2 in, 2 out]
                    n213 = property on="ReadMeasFromEEProm" class="Bool"("Disabled"=w399) -> ()  [unwired: 2 in, 2 out]
                    n214 = property on="StartMeasurement" class="Bool"("Disabled"=w399) -> ()  [unwired: 2 in, 2 out]
                    n215 = property on="DigitalIO" class="Bool"("Disabled"=w399) -> ()  [unwired: 2 in, 2 out]
                    n216 = property on="AnalogIO" class="Bool"("Disabled"=w399) -> ()  [unwired: 2 in, 2 out]
                  }
                }
              }
              event "StopMeasurement": Value Change {
                w401 = u8 0 ("Disabled")
                n217 = event-data() -> ()  [unwired: 1 in, 6 out]
                n218 = local read "a_hDevice"() -> (w400:i32)
                n219 = property on="StartMeasurement" class="Bool"("Disabled"=w401) -> ()  [unwired: 2 in, 2 out]
                n220 = property on="AnalogIO" class="Bool"("Disabled"=w401) -> ()  [unwired: 2 in, 2 out]
                n221 = property on="DigitalIO" class="Bool"("Disabled"=w401) -> ()  [unwired: 2 in, 2 out]
                n222 = property on="ReadMeasFromEEProm" class="Bool"("Disabled"=w401) -> ()  [unwired: 2 in, 2 out]
                n223 = property on="WriteMeasToEEProm" class="Bool"("Disabled"=w401) -> ()  [unwired: 2 in, 2 out]
                n224 = call "AVS_StopMeasure.vi"("a_hDevice"=w400) -> ()  [unwired: 14 in, 1 out]
              }
              event "Exit": Value Change {
                n225 = event-data() -> ()  [unwired: 1 in, 6 out]
              }
            }
            n226 = call "AVS_PollScan.vi"("a_hDevice"=w109) -> ("Output Value"=w108:i32)  [unwired: 8 in]
            n227 = Less Than 0?(x=w108) -> (x < 0?=w110:bool)
            n228 = case shown="True" w110 {
              tunnel: w108 -> [_ w164]
              frame False {
              }
              frame True {
                n229 = Number To Decimal String(number=w164) -> (decimal integer string=w163:string)  [unwired: 1 in]
                n230 = Concatenate Strings("Error code: ", w163) -> (w166:string)
                n231 = local write "Status"(w166) -> ()
              }
            }
            n232 = case shown="1" w108 {
              tunnel: [w112 w114] -> w106
              tunnel: w105 -> [w112 w113]
              frame 0, Default {
              }
              frame 1 {
                n233 = stacked-sequence {
                  seq-local: [_ w141 _] -> [_ _ w149]
                  tunnel: [_ w135 _] -> w118
                  tunnel: [w124 _ _] -> w115
                  tunnel: [_ w137 _] -> w114
                  tunnel: w113 -> [_ w136 _]
                  frame #0 {
                    n234 = local read "StopPixel"() -> (w122:u16)
                    n235 = local read "StartPixel"() -> (w121:u16)
                    n236 = local read "a_hDevice"() -> (w128:i32)
                    n237 = Subtract(x=w122, y=w121) -> (x-y=w120:u16)
                    n238 = local read "StartPixel"() -> (w123:u16)
                    n239 = Initialize Array(0.0, 4096 ("dimension size")) -> (w126:dbl[])
                    n240 = call "AVS_GetLambda.vi"("a_hDevice"=w128, "a_pWaveLength"=w126) -> ("a_pWaveLength"=w125:dbl[])  [unwired: 12 in, 1 out]
                    n241 = Array Subset(array=w125, index=w123, length=w120) -> (w124:dbl[])
                  }
                  frame #1 {
                    # "Returns the values for each pixel"
                    n242 = local read "StopPixel"() -> (w132:u16)
                    n243 = local read "StartPixel"() -> (w131:u16)
                    n244 = local read "a_hDevice"() -> (w140:i32)
                    n245 = local read "PerformedScans"() -> (w147:dbl)
                    n246 = Subtract(x=w132, y=w131) -> (x-y=w130:u16)
                    n247 = Initialize Array(0.0 ("element"), 4096 ("dimension size")) -> (w145:dbl[])
                    n248 = call "AVS_GetScopeData.vi"("a_hDevice"=w140, "a_pTimeLabel"=u32 0, "a_pSpectrum"=w145) -> ("a_pTimeLabel"=w137:u32, "a_pSpectrum"=w134:dbl[])  [unwired: 10 in, 1 out]
                    n249 = Array Subset(array=w134, index=0, length=w130) -> (w135:dbl[])
                    n250 = Increment(x=w147) -> (x+1=w148:dbl)
                    n251 = local write "Status"("Meas.Status: success" ("Status")) -> ()
                    n252 = local write "PerformedScans"(w148) -> ()
                    n253 = Subtract(x=w137, y=w136) -> (x-y=w138:u32)
                    n254 = Divide(x=w138, y=u32 100) -> (x/y=w141:dbl)
                  }
                  frame #2 {
                    n255 = Tick Count (ms)() -> (millisecond timer value=w161:u32)
                    n256 = local read "StartTime"() -> (w160:u32)
                    n257 = local read "PerformedScans"() -> (w151:dbl)
                    n258 = local read "NrOfScans"() -> (w152:i16)
                    n259 = Subtract(x=w161, y=w160) -> (x-y=w158:u32)
                    n260 = Equal?(x=w151, y=w152) -> (x = y?=w150:bool)
                    n261 = Divide(x=w158, y=u32 1000) -> (x/y=→"TotalTime":dbl)
                    n262 = Divide(x=w158, y=w151) -> (x/y=w155:dbl)
                    "AvgTimePerScan" <- w155
                    n263 = Less Or Equal?(x=w151, y=1.0 ("x")) -> (x <= y?=w157:bool)
                    n264 = case shown="True" w150 {
                      frame False {
                      }
                      frame True {
                        n265 = property on="StartMeasurement" class="Bool"("Disabled"=u8 0) -> ()  [unwired: 2 in, 2 out]
                      }
                    }
                    n266 = Select(t=w155, s=w157, f=w149) -> (s? t:f=→"LastScanTime":dbl)
                  }
                }
                n267 = call "Convert to Dynamic Data2"("Array"=w118) -> ("Dynamic Data Type"=w117:dynamicdata)  [unwired: 3 in]
                n268 = call "Convert to Dynamic Data"("Array"=w115) -> ("Dynamic Data Type"=w116:dynamicdata)  [unwired: 3 in]
                n269 = call "Build XY Graph"("Y Input"=w117, "X Input"=w116) -> ("XY Graph"=→"XY Graph":cluster{"Y":dbl[], "Y":dbl[]}[])  [unwired: 8 in, 1 out]
              }
            }
          }
        }
        frame #2 {
          n270 = flat-sequence {
            frame #0 {
              n271 = local read "a_hDevice"() -> (w403:i32)
              n272 = property on="StartMeasurement" class="Bool"("Disabled"=u8 0) -> ()  [unwired: 2 in, 2 out]
              n273 = call "AVS_StopMeasure.vi"("a_hDevice"=w403) -> ()  [unwired: 14 in, 1 out]
            }
            frame #1 {
              n274 = local read "a_hDevice"() -> (w405:i32)
              n275 = call "AVS_Deactivate.vi"("a_hHandle"=w405) -> ()  [unwired: 14 in, 1 out]
            }
            frame #2 {
              n276 = call "AVS_Done.vi"() -> ()  [unwired: 19 in, 1 out]
            }
          }
        }
      }
    }
  }
